vi "CollectData.vi"(8 "error in (no error)":errorcluster, 11 "NI Card in":refnum<class "NI Card.lvclass">) -> (0 "error out":errorcluster, 3 "NI Card out":refnum<class "NI Card.lvclass">)   [LabVIEW 2013, in "NI Card.lvclass"]
uses:
  NI Card.lvclass
  Device/Device.lvclass
  NI Card.lvclass/NI Card.ctl
  SetListPrefs/SetListPrefs.lvclass/SetListPrefs.ctl
  <vilib>/DAQmx/read.llb/DAQmx Read (Analog 1D DBL NChan 1Samp).vi
  <vilib>/DAQmx/read.llb/DAQmx Read (Analog 1D Wfm NChan NSamp).vi
  Globals/PrefsGlobal.vi
  <vilib>/DAQmx/miscellaneous.llb/DAQmx Fill In Error Info.vi
  <vilib>/Waveform/WDTOps.llb/WDT Append Waveforms DBL.vi
  SetListPrefs/SetListPrefs.lvclass
  <resource>/objmgr/daqmx.rc
panel:
  out "data":waveform(dbl)[](graph)
  out "First Data Point":dbl[](array[numeric]) format="%0.2f"
  out "Number of points read":i32[](array[numeric])
  out "AI Data":cluster{dbl[], "Y":dbl[], "String":string}[](array[cluster])
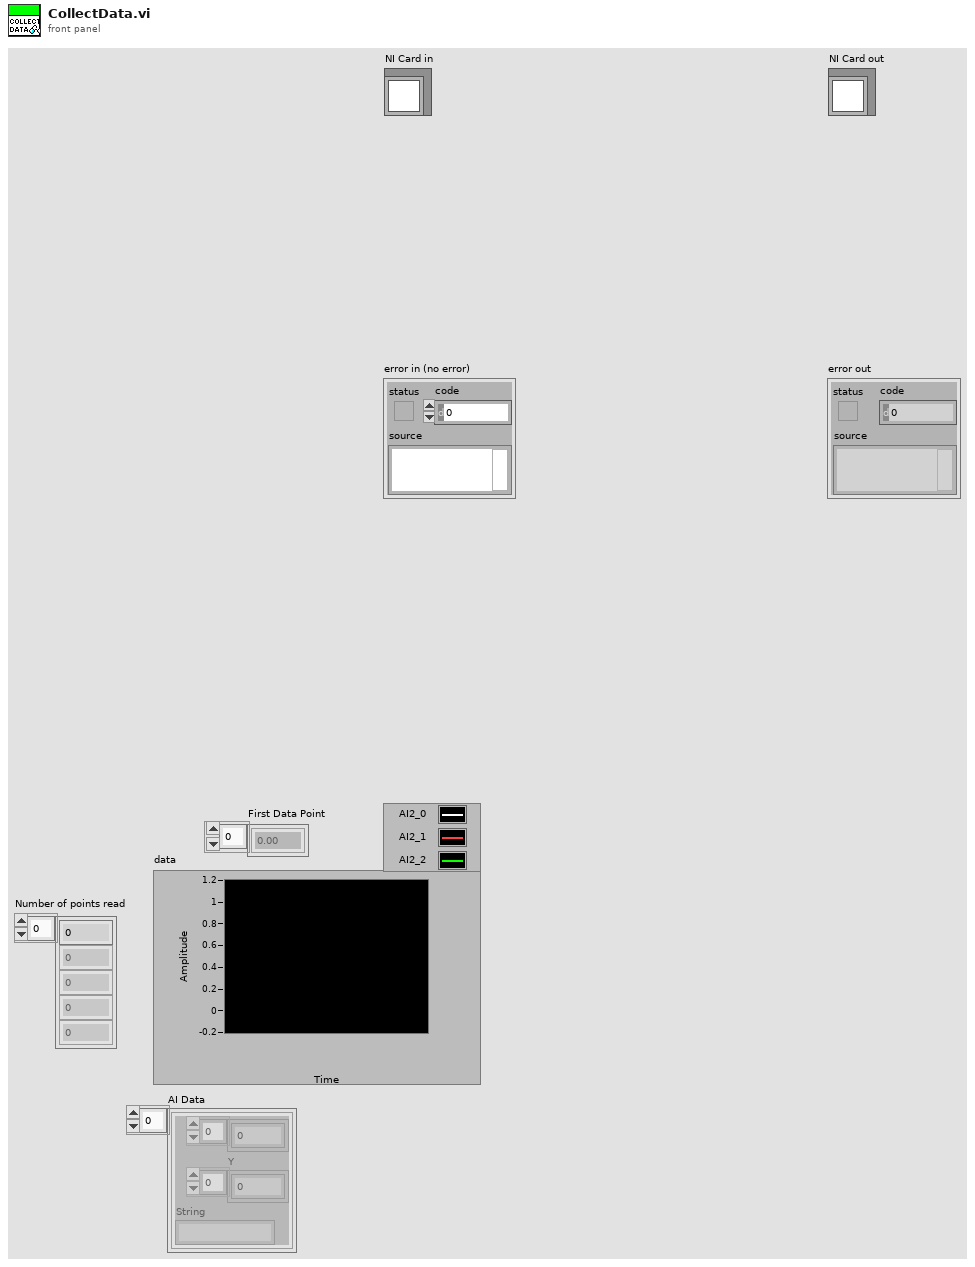
[diagram p1: front panel]
types:
  T1 = cluster{"DAQmx Global Channel":refnum<k21>, "String":string}[]
  T2 = typedef "NI Card.lvclass/AI_Data.ctl" = cluster{"t":dbl[], "y":dbl[], "Channel Name":string}
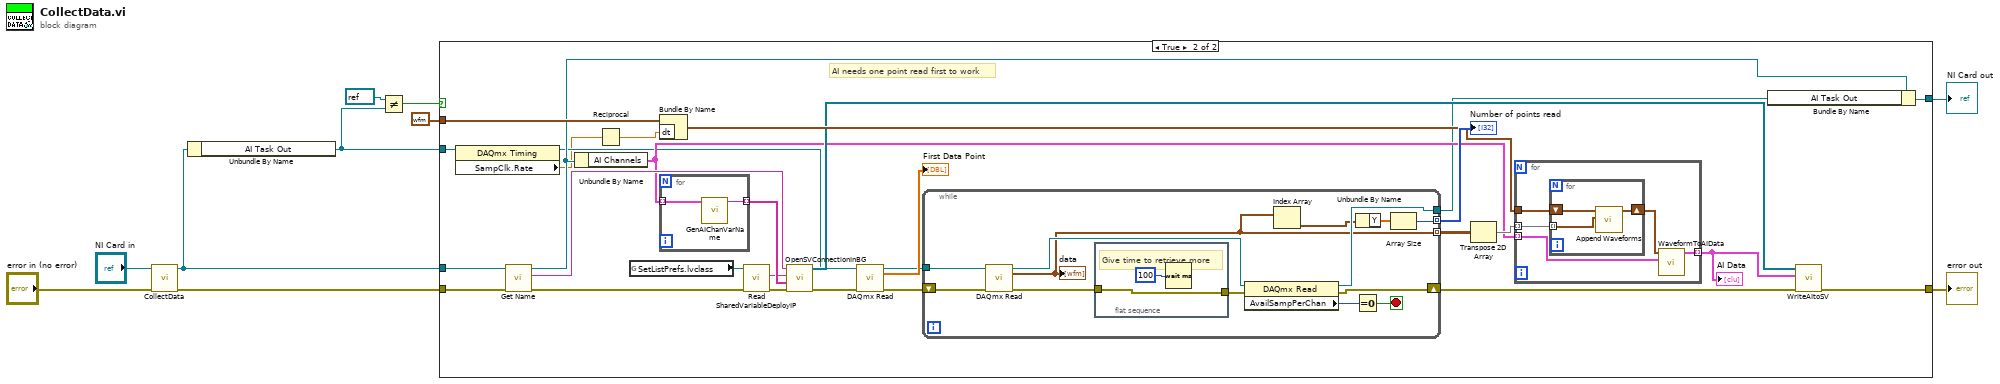
[diagram p0: block diagram]
diagram:
  n1 = call-parent "CollectData.vi"("error in (no error)"="error in (no error)", "Device in"="NI Card in") -> ("error out"=w4:errorcluster, "Device out"=w3:refnum<class "NI Card.lvclass">)  [unwired: 8 in]
  n2 = Unbundle By Name(w3) -> ("AI Task Out"=w7:refnum<k21>)
  n3 = Not Equal?(x=refnum<k21> refnum ("task out"), y=w7) -> (x != y?=w6:bool)
  n4 = case shown="True" w6 {
    tunnel: w7 -> [_ w15]
    tunnel: w4 -> [w12 w33]
    tunnel: [w12 w24] -> w2
    tunnel: waveform(dbl) {"t0"=timestamp(0 s since 1904-01-01), "dt"=0.001, "Y"=[]} ("Waveform") -> [_ w37]
    tunnel: w3 -> [w11 w34]
    tunnel: [w11 w20] -> w1
    frame False {
    }
    frame True {
      # "AI needs one point read first to work"
      n5 = property class="DAQmx Timing"(reference=w15) -> (reference out=w14:refnum<k21>, "SampClk.Rate"=w13:dbl)  [unwired: 1 in, 1 out]
      n6 = call-dynamic "Get Name.vi"("error in (no error)"=w33, "Device in"=w34) -> ("error out"=w25:errorcluster, "Name"=w35:string, "Device out"=w22:refnum<class "NI Card.lvclass">)  [unwired: 7 in]
      n7 = Unbundle By Name(w22) -> ("AI Channels"=w30:T1)
      n8 = Reciprocal(x=w13) -> (1/x=w36:dbl)
      n9 = global read "PrefsGlobal.vi" "SetListPrefs.lvclass"() -> (w28:refnum<class "SetListPrefs.lvclass">)
      n10 = Bundle By Name(cluster=w37, "dt"=w36) -> (w38:waveform(dbl))
      n11 = for {
        tunnel: [w43] -> w32 mode=indexing
        tunnel: w30 -> [w42] mode=indexing
        n12 = call "GenAIChanVarName.vi"("AI Channel"=w42) -> ("Channel Variable Name"=w43:string)  [unwired: 4 in]
      }
      n13 = call "Read SharedVariableDeployIP.vi"("error in (no error)"=w25, "SetListPrefs in"=w28) -> ("error out"=w26:errorcluster, "SharedVariableDeployIP"=w27:string)  [unwired: 7 in, 1 out]
      n14 = call "OpenSVConnectionInBG.vi"("error in (no error)"=w26, "ChannelNames"=w32, "Target IP"=w27, "DeviceName"=w35) -> ("error out"=w16:errorcluster, "SharedVariableRefnums"=w31:refnum<k21>[])  [unwired: 6 in]
      n15 = call-poly <vilib>:"DAQmx Read.vi"("task/channels in"=w14, "error in"=w16) -> ("task out"=w17:refnum<k21>, "data"=→"First Data Point":dbl[], "error out"=w18:errorcluster)  [unwired: 11 out]
      n16 = while {
        tunnel: w17 -> [w53]
        tunnel: [w63] -> w41 mode=indexing
        tunnel: [w60] -> w21
        tunnel: [w56] -> w40 mode=indexing
        shift-right: [w59] -> w23
        shift-left: w18 -> [w52]
        stop <- w62 stop-if-true
        n17 = call-poly <vilib>:"DAQmx Read.vi"("task/channels in"=w53, "error in"=w52) -> ("task out"=w61:refnum<k21>, "data"=w56:waveform(dbl)[], "error out"=w55:errorcluster)  [unwired: 1 in, 10 out]
        "data" <- w56
        n18 = flat-sequence {
          tunnel: w55 -> [w65]
          tunnel: [w65] -> w54
          frame #0 {
            # "Give time to retrieve more"
            n19 = Wait (ms)(milliseconds to wait=u32 100) -> ()  [unwired: 1 out]
          }
        }
        n20 = property class="DAQmx Read"(reference=w61, error in=w54) -> (reference out=w60:refnum<k21>, error out=w59:errorcluster, "AvailSampPerChan"=w58:u32)
        n21 = Index Array(array=w56) -> (element=w57:waveform(dbl))  [unwired: 1 in]
        n22 = Equal To 0?(x=w58) -> (x = 0?=w62:bool)
        n23 = Unbundle By Name(w57) -> ("Y"=w64:dbl[])
        n24 = Array Size(array=w64) -> (size(s)=w63:i32)
      }
      "Number of points read" <- w41
      n25 = Transpose 2D Array(2D array=w40) -> (transposed array=w39:waveform(dbl)[][])
      n26 = for {
        tunnel: w39 -> [w47] mode=indexing
        tunnel: w38 -> [w48]
        tunnel: w30 -> [w45] mode=indexing
        tunnel: [w44] -> w29 mode=indexing
        n27 = for {
          tunnel: w47 -> [w49] mode=indexing
          shift-right: [w51] -> w46
          shift-left: w48 -> [w50]
          n28 = call-poly <vilib>:"Append Waveforms.vi"("waveform B"=w49, "waveform A"=w50) -> ("waveform out"=w51:waveform(dbl))  [unwired: 1 in, 8 out]
        }
        n29 = call "WaveformToAIData.vi"("AI Channel"=w45, "AI Waveform"=w46) -> ("AI Data"=w44:T2)  [unwired: 8 in, 1 out]
      }
      "AI Data" <- w29
      n30 = Bundle By Name(cluster=w22, "AI Task Out"=w21) -> (w20:refnum<class "NI Card.lvclass">)
      n31 = call "WriteAItoSV.vi"("error in (no error)"=w23, "AI Data"=w29, "SharedVariableRefnums"=w31) -> ("error out"=w24:errorcluster)  [unwired: 8 in]
    }
  }
  "error out" <- w2
  "NI Card out" <- w1
